vi "Read Waveform (Multiple).vi"(8 "error in (no error)":errorcluster, 9 "Maximum Time (10000 ms)":u32=10000, 10 "Channels":u16[](array[ring])=[1, 2] items=["Channel 1"=1, "Channel 2"=2, "Channel 3"=3, "Channel 4"=4], 11 "VISA resource name":refnum<visa-resource-name>) -> (0 "error out":errorcluster, 2 "Waveform Data":waveform(dbl)[](graph), 3 "VISA resource name out":refnum<visa-resource-name>)   [LabVIEW 2011, in "Agilent DSO1000 Series.lvlib"]
doc: "Initiates an acquisition on all channels that you enabled with the Configure Channel VI. The VI waits for the acquisition to complete and returns the waveform for the <B>Source Channel</B> you specified. If the oscilloscope did not complete the acquisition within the time period you specify with the <B>Timeout</B> control, the VI returns a timeout error. A common cause for a timeout error is the acquisition was not triggered. For example, the trigger level is out of range of the waveform. \n\n<B>Note:</B> If your instrument does not support auto compensation for probe attenuation, you may need to adjust the scaling of the waveform data accordingly. This is handled automatically in the Configure Channel VI or can be done manually by multiplying the waveform data by the probe attenuation."
uses:
  <instrlib>/Agilent DSO1000 Series/Agilent DSO1000 Series.lvlib
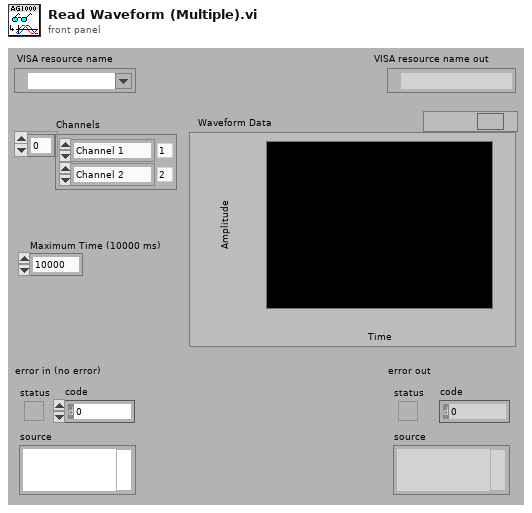
[diagram p1: front panel]
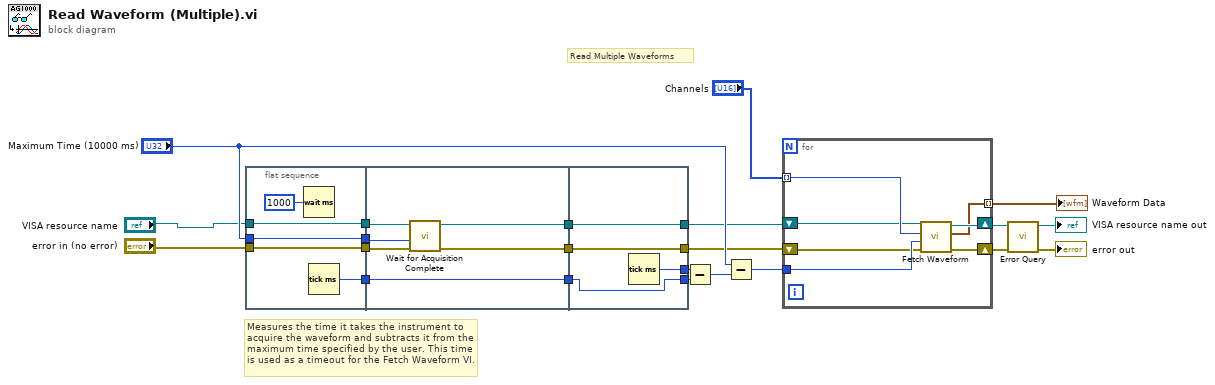
[diagram p0: block diagram]
diagram:
  # "Read Multiple Waveforms"
  # "Measures the time it takes the instrument to acquire the waveform and subtracts it from the maximum time specified by the user. This time is used as a timeout for the Fetch Waveform VI."
  n1 = flat-sequence {
    tunnel: "VISA resource name" -> [w26]
    tunnel: [w26] -> w11
    tunnel: "error in (no error)" -> [w25]
    tunnel: [w25] -> w10
    tunnel: "Maximum Time (10000 ms)" -> [w24]
    tunnel: [w24] -> w9
    tunnel: [w27] -> w8
    tunnel: w11 -> [w33]
    tunnel: [w32] -> w7
    tunnel: w10 -> [w31]
    tunnel: [w30] -> w6
    tunnel: w9 -> [w29]
    tunnel: w8 -> [w28]
    tunnel: [w28] -> w5
    tunnel: [w36] -> w4
    tunnel: w7 -> [w36]
    tunnel: [w35] -> w3
    tunnel: w6 -> [w35]
    tunnel: [w34] -> w15
    tunnel: w5 -> [w34]
    tunnel: [w37] -> w14
    frame #0 {
      n2 = Wait (ms)(milliseconds to wait=u32 1000) -> ()  [unwired: 1 out]
      n3 = Tick Count (ms)() -> (millisecond timer value=w27:u32)
    }
    frame #1 {
      n4 = call <instrlib>:"Wait for Acquisition Complete.vi"("error in (no error)"=w31, "Maximum Time (10000 ms)"=w29, "VISA resource name"=w33) -> ("error out"=w30:errorcluster, "VISA resource name out"=w32:refnum<visa-resource-name>)  [unwired: 7 in]
    }
    frame #2 {
      n5 = Tick Count (ms)() -> (millisecond timer value=w37:u32)
    }
  }
  n6 = Subtract(x=w14, y=w15) -> (x-y=w16:u32)
  n7 = Subtract(x="Maximum Time (10000 ms)", y=w16) -> (x-y=w13:u32)
  n8 = for {
    shift-right: [w43] -> w19
    shift-left: w3 -> [w38]
    tunnel: "Channels" -> [w42] mode=indexing
    tunnel: [w41] -> w17 mode=indexing
    shift-right: [w44] -> w20
    shift-left: w4 -> [w39]
    tunnel: w13 -> [w40]
    n9 = call <instrlib>:"Fetch Waveform.vi"("error in (no error)"=w38, "Maximum Time (10000 ms)"=w40, "Channel (1: Channel 1)"=w42, "VISA resource name"=w39) -> ("error out"=w43:errorcluster, "Waveform Data"=w41:waveform(dbl), "VISA resource name out"=w44:refnum<visa-resource-name>)  [unwired: 5 in]
  }
  "Waveform Data" <- w17
  n10 = call <instrlib>:"Error Query.vi"("error in (no error)"=w19, "VISA resource name"=w20) -> ("error out"=→"error out":errorcluster, "VISA resource name out"=→"VISA resource name out":refnum<visa-resource-name>)  [unwired: 6 in, 2 out]
